vi "View Error Log Mode Functional Global.vi"(8 "Error In":errorcluster) -> (0 "Error Out":errorcluster)   [LabVIEW 2012, in "OpenCLV x64.lvlib"]
doc: "Shows the errors that have occured in a since starting the program."
uses:
  OpenCLV x64.lvlib
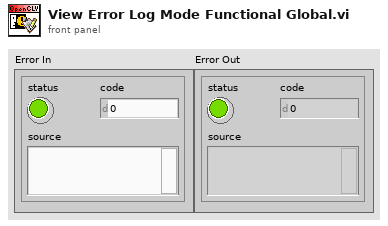
[diagram p1: front panel]
types:
  T1 = enum16{"Initialize", "Add Error", "View Error Log", "Save Error Log", "Set Verbose Mode", "Set Quite Mode"}
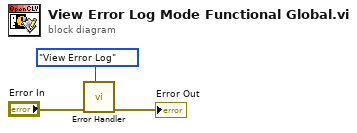
[diagram p0: block diagram]
diagram:
  n1 = call "Error Handler.vi"("Error Handler States"=T1."View Error Log", "Error In"="Error In") -> ("Error Out"=→"Error Out":errorcluster)  [unwired: 9 in]
